vi "Config String to Config.vi"(8 "error in":errorcluster, 11 "Input String":string) -> (0 "error out":errorcluster, 3 "Config Cluster out":T1)   [LabVIEW 2017]
uses:
  Config Cluster.ctl
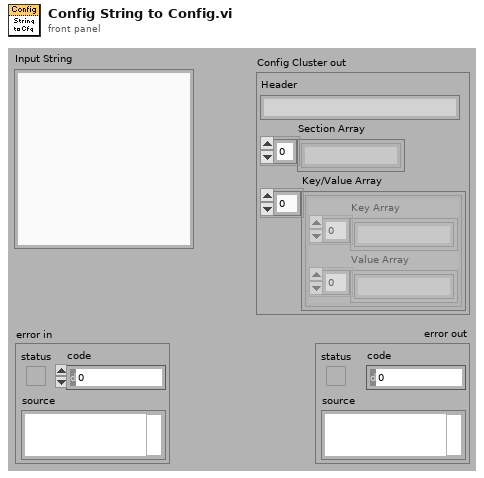
[diagram p1: front panel]
types:
  T1 = typedef "Config Cluster.ctl" = cluster{"Header":string, "Section Array":string[], "Key/Value Array":cluster{"Key Array":string[], "Value Array":string[]}[]}
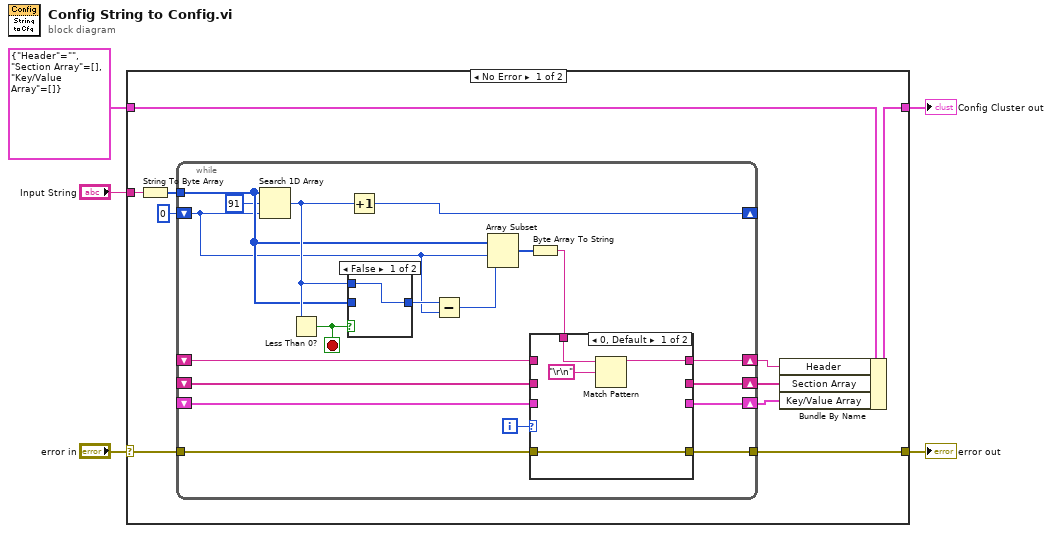
[diagram p0: block diagram]
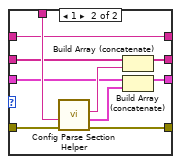
[diagram p2: hidden frame]
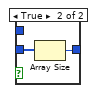
[diagram p3: hidden frame]
diagram:
  n1 = case shown="No Error" "error in" {
    selector: "error in" -> [w10 w53]
    tunnel: [w13 w52] -> w5
    tunnel: [w12 w53] -> w4
    tunnel: "Input String" -> [w11 _]
    tunnel: T1 {"Header"="", "Section Array"=[], "Key/Value Array"=[]} ("Config File.lvclass 2 out") -> [w9 w52]
    frame No Error {
      n2 = String To Byte Array(string=w11) -> (unsigned byte array=w15:u8[])
      n3 = while {
        tunnel: w15 -> [w22]
        shift-right: [w20] -> _
        shift-left: 0 -> [w19]
        tunnel: [w27] -> w12
        tunnel: w10 -> [w28]
        shift-right: [w26] -> w8
        shift-left: _ -> [w24]
        shift-right: [w25] -> w7
        shift-left: _ -> [w23]
        shift-right: [w17] -> w6
        shift-left: _ -> [w18]
        i -> [w16]
        stop <- w33 stop-if-true
        n4 = Search 1D Array(1D array=w22, element=u8 91, start index (0)=w19) -> (index of element=w30:i32)
        n5 = Less Than 0?(x=w30) -> (x < 0?=w33:bool)
        n6 = case shown="False" w33 {
          tunnel: w30 -> [w49 _]
          tunnel: [w49 w50] -> w31
          tunnel: w22 -> [_ w51]
          frame False {
          }
          frame True {
            n7 = Array Size(array=w51) -> (size(s)=w50:i32)
          }
        }
        n8 = Increment(x=w30) -> (x+1=w20:i32)
        n9 = Subtract(x=w31, y=w19) -> (x-y=w34:i32)
        n10 = Array Subset(array=w22, index=w19, length=w34) -> (w32:u8[])
        n11 = Byte Array To String(unsigned byte array=w32) -> (string=w29:string)
        n12 = case shown="0, Default" w16 {
          tunnel: w29 -> [w36 w48]
          tunnel: w28 -> [w38 w47]
          tunnel: [w38 w46] -> w27
          tunnel: [_ w44] -> w26
          tunnel: [_ w43] -> w25
          tunnel: w24 -> [_ w41]
          tunnel: w23 -> [_ w40]
          tunnel: w18 -> [_ w39]
          tunnel: [w35 w39] -> w17
          frame 0, Default {
            n13 = Match Pattern(string=w36, regular expression="\r\n") -> (before substring=w35:string)  [unwired: 1 in, 3 out]
          }
          frame 1 {
            n14 = call "Config Parse Section Helper.vi"("error in"=w47, "String In"=w48) -> ("error out"=w46:errorcluster, "Key/Value array"=w45:cluster{string[], string[]}, "Section Out"=w42:string)  [unwired: 7 in]
            n15 = Build Array (concatenate)(w41, w42) -> (w44:string[])
            n16 = Build Array (concatenate)(w40, w45) -> (w43:cluster{string[], string[]}[])
          }
        }
      }
      n17 = Bundle By Name(cluster=w9, "Header"=w6, "Section Array"=w8, "Key/Value Array"=w7) -> (w13:T1)
    }
    frame Error {
    }
  }
  "error out" <- w4
  "Config Cluster out" <- w5
